vi "PID_controller.vi"(1 "Error_Sum(k-1)":dbl, 3 "Error(k-1)":dbl, 4 "Ki":dbl, 5 "Kd":dbl, 6 "Kp":dbl, 7 "Error(k)":dbl) -> (0 "u(k)":dbl, 2 "Error_Sum(k)":dbl)   [LabVIEW 2019]
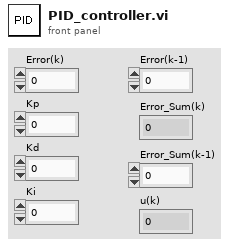
[diagram p1: front panel]
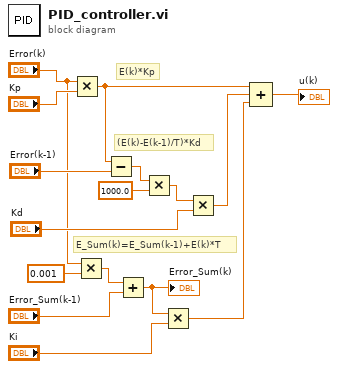
[diagram p0: block diagram]
diagram:
  # "E_Sum(k)=E_Sum(k-1)+E(k)*T"
  # "(E(k)-E(k-1)/T)*Kd"
  # "E(k)*Kp"
  n1 = Multiply(x="Error(k)", y="Kp") -> (x*y=w14:dbl)
  n2 = Multiply(x="Error(k)", y=0.001) -> (x*y=w5:dbl)
  n3 = Subtract(x=w14, y="Error(k-1)") -> (x-y=w12:dbl)
  n4 = Add(x=w5, y="Error_Sum(k-1)") -> (x+y=w1:dbl)
  "Error_Sum(k)" <- w1
  n5 = Multiply(x=w12, y=1000.0) -> (x*y=w10:dbl)
  n6 = Multiply(x=w1, y="Ki") -> (x*y=w2:dbl)
  n7 = Multiply(x=w10, y="Kd") -> (x*y=w8:dbl)
  n8 = Compound Arithmetic op=ADD(w14, w8, w2) -> (→"u(k)":dbl)
